vi "QTrkBuildLUTPlane.vi"(0 "QTrk Instance":T1, 5 "Bead images":sgl[][][](array[numeric]), 7 "flags":u32, 9 "plane":i32, 11 "error in (no error)":errorcluster) -> (4 "QTrk Instance":T1, 15 "error out":errorcluster)   [LabVIEW 2011]
uses:
  QTrkInstance.ctl
  QTrkDLL.vi
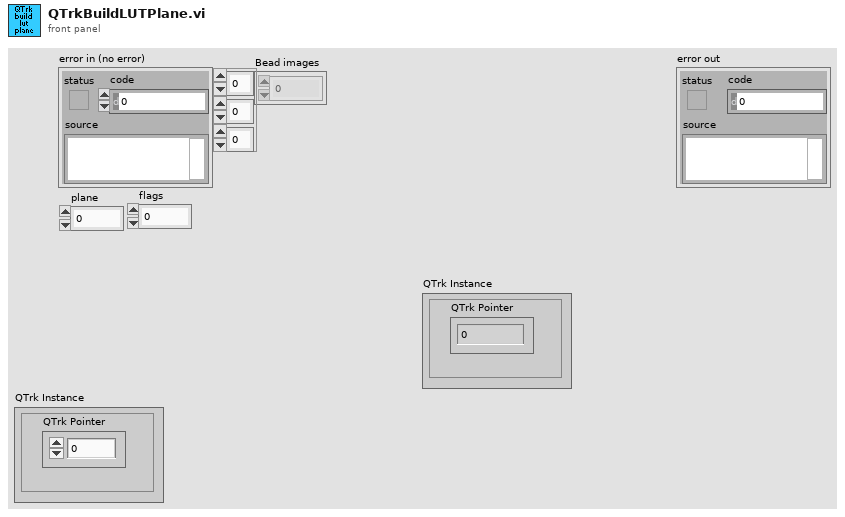
[diagram p1: front panel]
types:
  T1 = typedef "QTrkInstance.ctl" = cluster{"QTrk Pointer":u64}
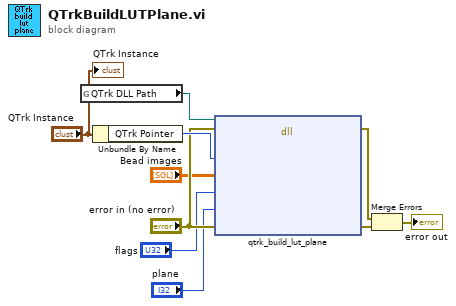
[diagram p0: block diagram]
diagram:
  n1 = global read "QTrkDLL.vi" "QTrk DLL Path"() -> (w8:path)
  n2 = Unbundle By Name("QTrk Instance") -> ("QTrk Pointer"=w9:u64)
  n3 = dll-call lib="D:/jcnossen1/cudaqi-tracker/bin/jtrk-labview.dll" fn="qtrk_build_lut_plane"(path in=w8, error in="error in (no error)", "tracker"=w9, "data"="Bead images", "flags"="flags", "plane"="plane", "error"="error in (no error)") -> (error out=w5:errorcluster, "error"=w6:errorcluster)  [unwired: 6 in, 1 out]
  n4 = Merge Errors(w5, w6) -> (→"error out":errorcluster)
  "QTrk Instance" <- "QTrk Instance"
